vi "Set Description.vi"(8 "error in (no error)":errorcluster, 10 "Description":string, 11 "CubeLogger in":refnum<class "CubeLogger.lvclass">) -> (0 "error out":errorcluster, 3 "CubeLogger out":refnum<class "CubeLogger.lvclass">)   [LabVIEW 2018, in "vis3d.lvlib" / "CubeLogger.lvclass"]
uses:
  CubeLogger.lvclass
  CubeLogger.lvclass/CubeLogger.ctl
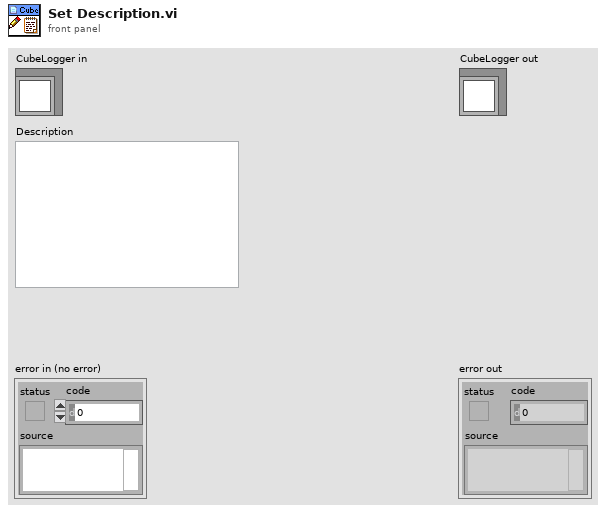
[diagram p1: front panel]
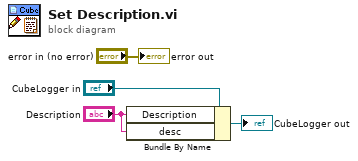
[diagram p0: block diagram]
diagram:
  n1 = Bundle By Name(cluster="CubeLogger in", "Description"="Description", "desc"="Description") -> (→"CubeLogger out":refnum<class "CubeLogger.lvclass">)
  "error out" <- "error in (no error)"
